vi "VI_RemoveBreakpoints_SSS_InternalFunctions.vi"() -> ()   [LabVIEW 2014]
panel:
  out "Remove Breakpoints Sum":u32
  out "All VI References":refnum<vi>[](array[refnum])
  out "Remove Breakpoints":u32
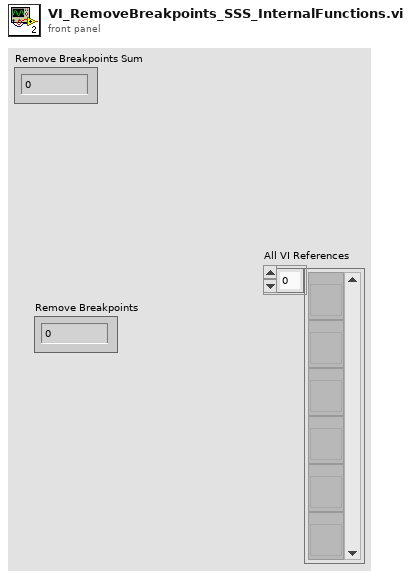
[diagram p1: front panel]
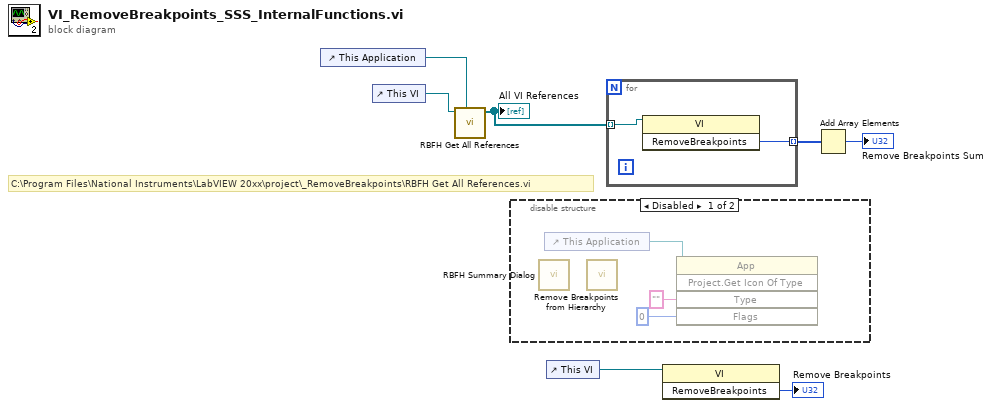
[diagram p0: block diagram]
diagram:
  # "C:\\Program Files\\National Instruments\\LabVIEW 20xx\\project\\_RemoveBreakpoints\\RBFH Get All References.vi"
  n1 = control-ref of="This Application"() -> (w5:refnum<vi>)
  n2 = control-ref of="This VI"() -> (w4:refnum<vi>)
  n3 = call "RBFH Get All References.vi"("Owning Application"=w5, "Main VI Refnum"=w4) -> ("All VI References"=w1:refnum<vi>[])  [unwired: 8 in, 1 out]
  "All VI References" <- w1
  n4 = disable-structure shown="Disabled" {
    frame Disabled {
      n5 = call "RBFH Summary Dialog.vi"() -> ()  [unwired: 12 in]
      n6 = control-ref of="This Application"() -> (w10:refnum<vi>)
      n7 = call "Remove Breakpoints from Hierarchy.vi"() -> ()  [unwired: 1 in]
      n8 = invoke class="App" method="Project.Get Icon Of Type"(reference=w10, "Type"="", "Flags"=0) -> ()  [unwired: 2 in, 5 out]
    }
    frame Enabled {
    }
  }
  n9 = control-ref of="This VI"() -> (w7:refnum<vi>)
  n10 = for {
    tunnel: [w12] -> w3 mode=indexing
    tunnel: w1 -> [w11] mode=indexing
    n11 = invoke class="VI" method="RemoveBreakpoints"(reference=w11) -> ("RemoveBreakpoints"=w12:u32)  [unwired: 2 in, 2 out]
  }
  n12 = invoke class="VI" method="RemoveBreakpoints"(reference=w7) -> ("RemoveBreakpoints"=→"Remove Breakpoints":u32)  [unwired: 2 in, 2 out]
  n13 = Add Array Elements(numeric array=w3) -> (sum=→"Remove Breakpoints Sum":u32)
